vi "WPI_AnalogChannelChannelCache.vi"(7 "Operation":T2, 8 "error in (no error)":errorcluster, 10 "Channel":T1=enum."AI 1") -> (0 "error out":errorcluster, 2 "Allocated?":bool, 3 "Allocated Channel":T1=enum."AI 1")   [LabVIEW 2017]
doc: "This software is licensed. Open the labview\\readme\\WPI Robotics Library Open Source License.txt file for more information."
uses:
  <vilib>/Rock Robotics/WPI/AnalogChannel/WPI_AnalogChannelChannelCacheOp.ctl
  <vilib>/Rock Robotics/SystemInterfaces/AI/FPGA_AIChannel.ctl
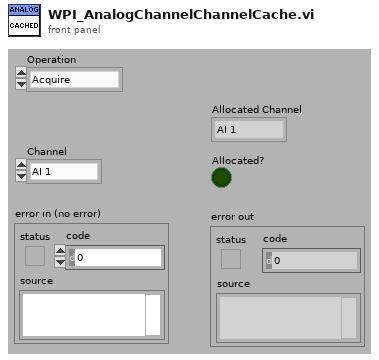
[diagram p1: front panel]
types:
  T1 = typedef "FPGA_AIChannel.ctl" = enum8{"AI 0", "AI 1", "AI 2", "AI 3", "AI MXP 0", "AI MXP 1", "AI MXP 2", "AI MXP 3", "Invalid"}
  T2 = typedef "WPI_AnalogChannelChannelCacheOp.ctl" = enum16{"Acquire", "Release", "Status"}
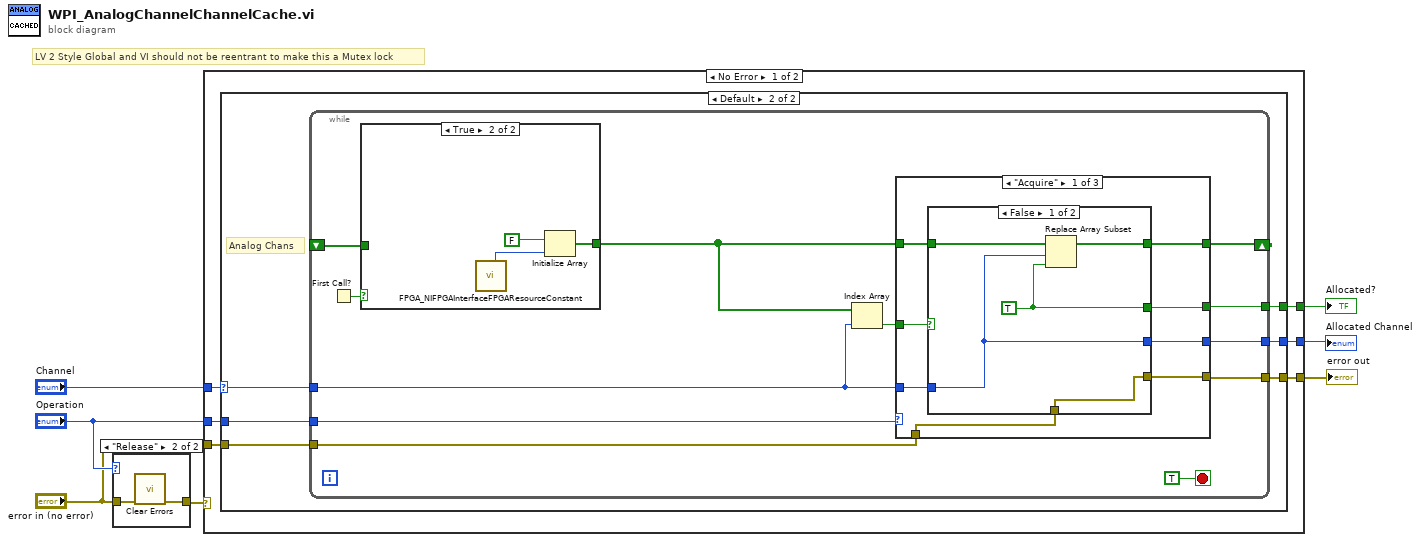
[diagram p0: block diagram]
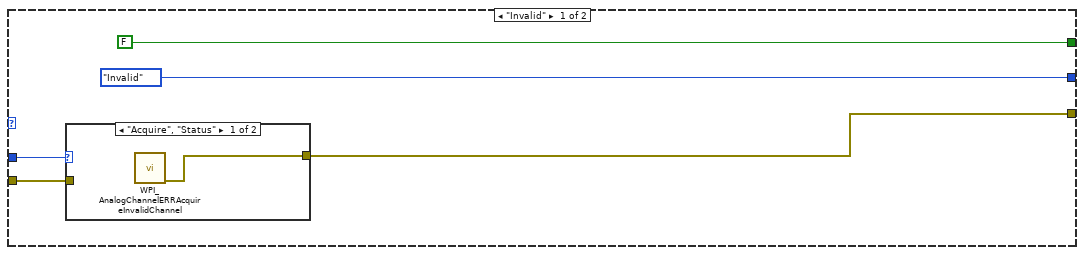
[diagram p3: hidden frame]
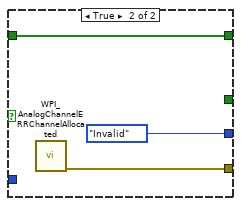
[diagram p5: hidden frame]
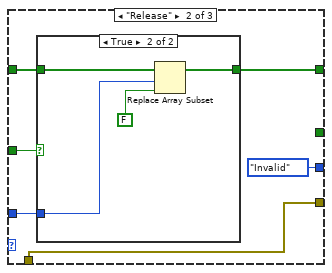
[diagram p6: hidden frame]
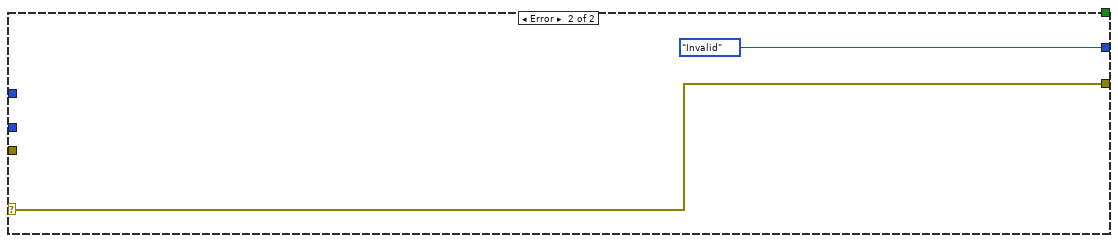
[diagram p10: hidden frame]
diagram:
  # "LV 2 Style Global and VI should not be reentrant to make this a Mutex lock"
  n1 = case shown="\"Release\"" "Operation" {
    tunnel: "error in (no error)" -> [w8 w10]
    tunnel: [w8 w9] -> w6
    frame "Acquire", Default {
    }
    frame "Release" {
      n2 = call <vilib>:"Clear Errors.vi"("error in (no error)"=w10) -> ("error out"=w9:errorcluster)  [unwired: 1 in, 5 out]
    }
  }
  n3 = case shown="No Error" w6 {
    selector: w6 -> [_ w78]
    tunnel: "Operation" -> [w16 _]
    tunnel: "Channel" -> [w15 _]
    tunnel: [w14 w78] -> w1
    tunnel: [w13 _] -> w5
    tunnel: [w12 FPGA_AIChannel."Invalid" ("Channel")] -> w4
    tunnel: "error in (no error)" -> [w11 _]
    frame No Error {
      n4 = case shown="Default" w15 {
        selector: w15 -> [_ w25]
        tunnel: w16 -> [w21 w29]
        tunnel: [w20 w28] -> w14
        tunnel: [FALSE ("new element/subarray") w27] -> w13
        tunnel: [FPGA_AIChannel."Invalid" ("Channel") w26] -> w12
        tunnel: w11 -> [w17 w24]
        frame "Invalid" {
          n5 = case shown="\"Acquire\", \"Status\"" w21 {
            tunnel: [w22 w23] -> w20
            tunnel: w17 -> [_ w23]
            frame "Acquire", "Status" {
              n6 = call <vilib>:"WPI_AnalogChannelERRAcquireInvalidChannel.vi"() -> ("error out"=w22:errorcluster)  [unwired: 11 in]
            }
            frame "Release" {
            }
          }
        }
        frame Default {
          # "Analog Chans"
          n7 = while {
            shift-right: [w38] -> _
            shift-left: _ -> [w40]
            tunnel: w29 -> [w39]
            tunnel: w25 -> [w34]
            tunnel: [w37] -> w28
            tunnel: [w36] -> w27
            tunnel: [w33] -> w26
            tunnel: w24 -> [w31]
            stop <- TRUE stop-if-true
            n8 = First Call?() -> (First Call?: T/F=w41:bool)
            n9 = case shown="True" w41 {
              tunnel: w40 -> [w73 _]
              tunnel: [w73 w75] -> w35
              frame False {
              }
              frame True {
                n10 = call <vilib>:"FPGA_NIFPGAInterfaceFPGAResourceConstant.vi"() -> ("NumberOfAIChannels"=w74:u8)  [unwired: 11 out]
                n11 = Initialize Array(FALSE, w74) -> (w75:bool[])
              }
            }
            n12 = Index Array(array=w35, index=w34) -> (element=w30:bool)
            n13 = case shown="\"Acquire\"" w39 {
              tunnel: w35 -> [w45 w63 w70]
              tunnel: [w49 w61 w70] -> w38
              tunnel: w34 -> [w48 w62 w72]
              tunnel: [w47 w58 w69] -> w37
              tunnel: [w46 _ w71] -> w36
              tunnel: w30 -> [w44 w60 w71]
              tunnel: [w43 FPGA_AIChannel."Invalid" ("Channel") w72] -> w33
              tunnel: w31 -> [w42 w58 w69]
              frame "Acquire" {
                n14 = case shown="False" w44 {
                  tunnel: w45 -> [w53 w57]
                  tunnel: [w52 w57] -> w49
                  tunnel: w48 -> [w51 _]
                  tunnel: [w50 w55] -> w47
                  tunnel: [w54 _] -> w46
                  tunnel: [w51 FPGA_AIChannel."Invalid" ("Channel")] -> w43
                  tunnel: w42 -> [w50 _]
                  frame False {
                    w54 = TRUE ("new element/subarray")
                    n15 = Replace Array Subset(array=w53, new element=w54, index=w51) -> (w52:bool[])
                  }
                  frame True {
                    n16 = call <vilib>:"WPI_AnalogChannelERRChannelAllocated.vi"() -> ("ERRChannelAllocated"=w55:errorcluster)  [unwired: 11 in]
                  }
                }
              }
              frame "Release" {
                n17 = case shown="True" w60 {
                  tunnel: w63 -> [w64 w68]
                  tunnel: w62 -> [_ w67]
                  tunnel: [w64 w66] -> w61
                  frame False {
                  }
                  frame True {
                    n18 = Replace Array Subset(array=w68, new element=FALSE ("new element/subarray"), index=w67) -> (w66:bool[])
                  }
                }
              }
              frame "Status" {
              }
            }
          }
        }
      }
    }
    frame Error {
    }
  }
  "error out" <- w1
  "Allocated?" <- w5
  "Allocated Channel" <- w4
